vi "Smart Open.vi"(7 "Allow multiple opens?":bool=TRUE, 8 "error in (no error)":errorcluster, 10 "Channel Names":tag[](array[tag])) -> (0 "error out":errorcluster, 3 "AudioIn (N Samples) Ref Out":T1)   [LabVIEW 2021, in "AudioIn Block.lvlib"]
doc: "Opens a reference to audio input block read channels. You must open a reference before you read values from the audio input block read channels."
uses:
  <vilib>/myRIO/Instrument Drivers/Onboard IO/AudioIn Block/AudioIn Block.lvlib
  <vilib>/myRIO/Common/Instrument Driver Framework/Utilities/typedefs/Hardware Version Enum.ctl
  <vilib>/myRIO/Common/Instrument Driver Framework/Utilities/typedefs/Generic FPGA Reference.ctl
  <vilib>/myRIO/Common/Instrument Driver Framework/Utilities/typedefs/myRIO v1.0 Reference.ctl
  <vilib>/myRIO/Common/Instrument Driver Framework/Utilities/typedefs/myRIO Generic Hardware Reference.ctl
  <vilib>/myRIO/Common/Instrument Driver Framework/myRIO v1.0/AudioIn Block/typedefs/AudioIn Block Channels Enum.ctl
  <vilib>/myRIO/Common/Instrument Driver Framework/myRIO v1.0/AudioIn Block/typedefs/AudioIn Block Channels List.ctl
  <vilib>/myRIO/Instrument Drivers/Onboard IO/AudioIn Block/typedefs/AudioIn Block Reference.ctl
  <vilib>/myRIO/Common/Instrument Driver Framework/Utilities/typedefs/Analog Scaling Constants.ctl
  <vilib>/myRIO/Instrument Drivers/Onboard IO/AudioIn Block/vis/myRIO AudioIn N Samples Open.xnode
  <vilib>/myRIO/Common/Instrument Driver Framework/myRIO v1.0/AudioIn Block/vis/myRIO v1.1 Open Throughput AudioIn (N Samples).vi
  <vilib>/userdefined/High Color/nirio_resource_hc.ctl
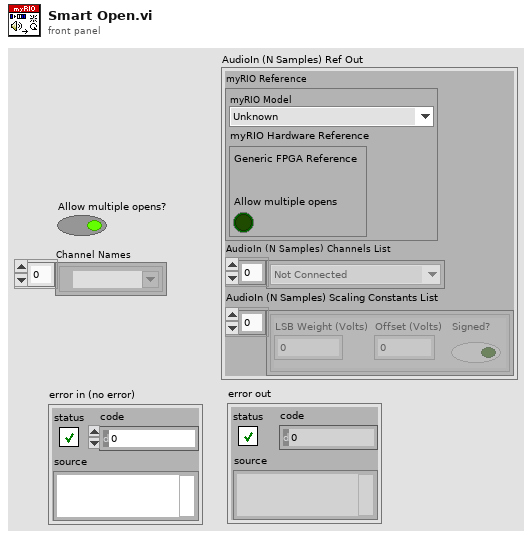
[diagram p1: front panel]
types:
  T1 = typedef "AudioIn Block.lvlib/AudioIn Block Reference.ctl" = cluster{"myRIO Reference":T2, "AudioIn (N Samples) Channels List":T6, "AudioIn (N Samples) Scaling Constants List":T8[]}
  T2 = typedef "myRIO Generic Hardware Reference.ctl" = cluster{"myRIO Model":T3, "myRIO Hardware Reference":T4}
  T3 = typedef "Hardware Version Enum.ctl" = enum16{"Unknown", "myRIO-1900", "myRIO-1950", "roboRIO", "NI ELVIS RIO CM", "ELVIS III"}
  T4 = typedef "myRIO v1.0 Reference.ctl" = cluster{"Generic FPGA Reference":T5, "Allow multiple opens":bool}
  T5 = typedef "Generic FPGA Reference.ctl" = refnum<k20>
  T6 = typedef "AudioIn Block Channels List.ctl" = T7[]
  T7 = typedef "AudioIn Block Channels Enum.ctl" = enum16{"Not Connected", "AudioIn/Left (N Samples)", "AudioIn/Right (N Samples)"}
  T8 = typedef "Analog Scaling Constants.ctl" = cluster{"LSB Weight (Volts)":dbl, "Offset (Volts)":dbl, "Signed?":bool}
  T9 = typedef "nirio_resource_hc.ctl" = tag
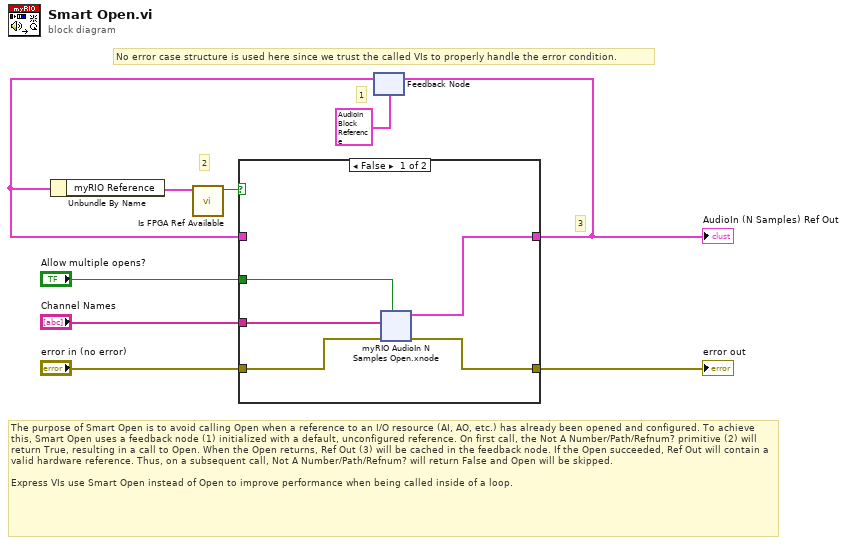
[diagram p0: block diagram]
diagram:
  # "No error case structure is used here since we trust the called VIs to properly handle the error condition."
  # "3"
  # "1"
  # "2"
  # "The purpose of Smart Open is to avoid calling Open when a reference to an I/O resource (AI, AO, etc.) has already been opened and configured. To achieve this, Smart Open uses a feedback node (1) initialized with a default, unconfigured reference. On first call, the Not A Number/Path/Refnum? primitive (2) will return True, resulting in a call to Open. When the Open returns, Ref Out (3) will be cached in the feedback node. If the Open succeeded, Ref Out will contain a valid hardware reference. Thus, on a subsequent call, Not A Number/Path/Refnum? will return False and Open will be skipped.\n\t\nExpress VIs use Smart Open instead of Open to improve performance when being called inside of a loop."
  n1 = feedback #1(T1 {"myRIO Reference"={"myRIO Model"=enum."Unknown", "myRIO Hardware Reference"={"Generic FPGA Reference"=refnum, "Allow multiple opens"=FALSE}}, "AudioIn (N Samples) Channels List"=[], "AudioIn (N Samples) Scaling Constants List"=[]} ("AI (N Samples) Read Ref Out")) -> (w9:T1)
  n2 = Unbundle By Name(w9) -> ("myRIO Reference"=w1:T2)
  n3 = call <vilib>:"Is FPGA Ref Available.vi"("myRIO Reference"=w1) -> ("Is Available?"=w8:bool)  [unwired: 10 in]
  n4 = case shown="False" w8 {
    tunnel: "error in (no error)" -> [w13 w33]
    tunnel: [w12 w34] -> w3
    tunnel: [w11 w33] -> w5
    tunnel: w9 -> [_ w34]
    tunnel: "Channel Names" -> [w14 _]
    tunnel: "Allow multiple opens?" -> [w10 _]
    frame False {
      n5 = xnode "myRIO AudioIn N Samples Open.xnode"("error in (no error)"=w13, "Allow multiple opens?"=w10, "Channel Names"=w14) -> ("error out"=w11:errorcluster, "AudioIn (N Samples) Ref Out"=w12:T1)
    }
    frame True {
    }
  }
  "AudioIn (N Samples) Ref Out" <- w3
  "error out" <- w5
  n6 = feedback-in #1(w3) -> ()
